vi "Column Headers.vi"(9 "View表":string="[v_runcondition]", 11 "DBLink":string="Driver={ODBC Driver 17 for SQL Server};Server=localhost\\SQLEXPRESS;Database=ZDX201;UID=labview;PWD=Dsa@54137926") -> (1 "資料表欄位名稱":string[](array[string]), 3 "欄位數":i32)   [LabVIEW 2019]
doc: "This VI was put together by AE Steve Karcher with AE Specialist Jonathan Cotton's help."
uses:
  <vilib>/addons/database/Auxilliary.llb/DB Tools Column Info.ctl
  <vilib>/addons/database/Auxilliary.llb/DB Tools DataTypes.ctl
  <vilib>/addons/database/Connection.llb/DB Tools Open Connec (String).vi
  <vilib>/addons/database/Connection.llb/Conn Execute.vi
  <vilib>/addons/database/Recordset.llb/Rec Destroy - Connection.vi
  <vilib>/addons/database/NI_Database_API.lvlib
  <vilib>/addons/database/Recordset.llb/Rec Fetch Recordset Data (R).vi
panel:
  in  "error in (no error)":errorcluster
  out "recordset data":variant[][](array[variant])
  out "error out":errorcluster
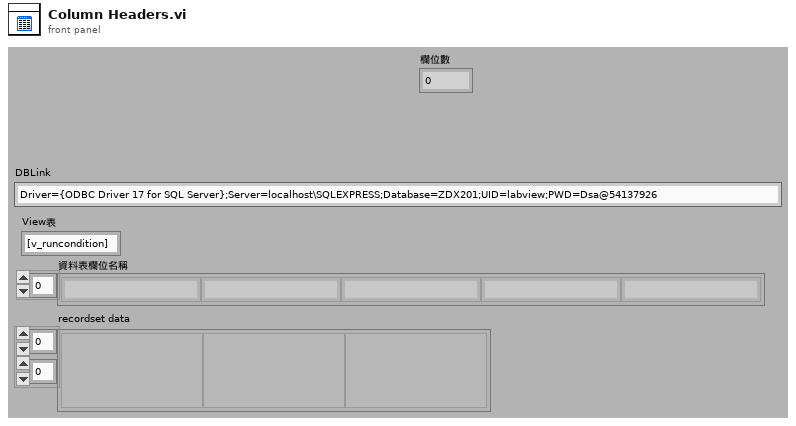
[diagram p1: front panel]
types:
  T1 = cluster{"String":string, "Numeric":i32, "Numeric 2":dbl}
  T2 = typedef "NI_Database_API.lvlib/DB Tools Column Info.ctl" = cluster{"column name":string, "data type":T3, "size":i32, "allow null?":bool}
  T3 = typedef "NI_Database_API.lvlib/DB Tools DataTypes.ctl" = enum16{"String", "Long (I32)", "Single (SGL)", "Double (DBL)", "Date/Time", "Binary"}
  T4 = typedef "NI_Database_API.lvlib/Conn ObjectReference.ctl" = refnum<k1>
  T5 = typedef "NI_Database_API.lvlib/Rec ObjectReference.ctl" = refnum<k1>
  T6 = typedef "NI_Database_API.lvlib/Rec DataMembers.ctl" = cluster{"ADODB._Recordset":refnum<k7>, "Connection":T4}
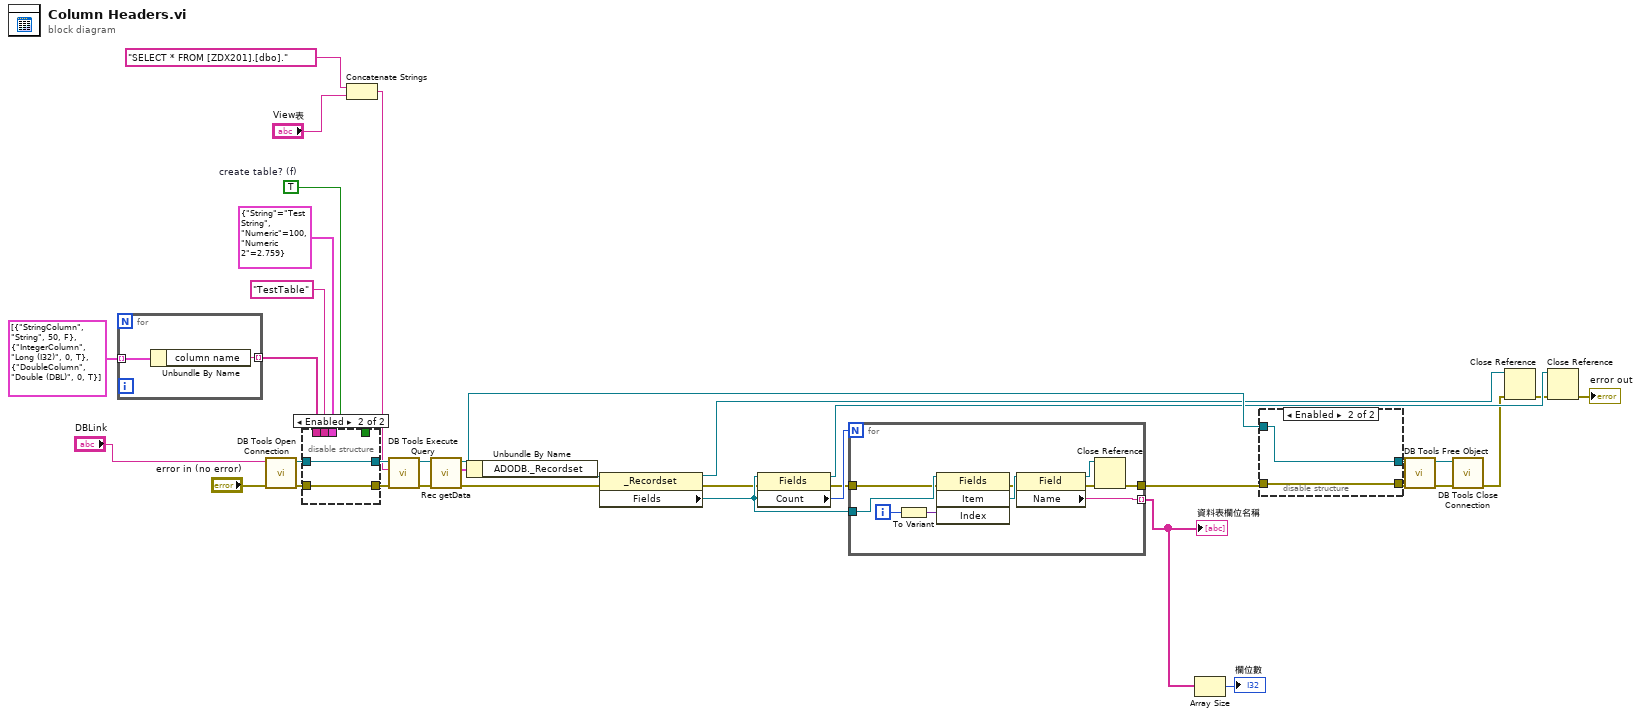
[diagram p0: block diagram]
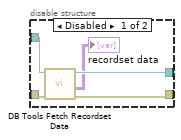
[diagram p2: hidden frame]
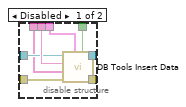
[diagram p3: hidden frame]
diagram:
  w27 = TRUE  # create table? (f)
  n1 = for {
    tunnel: T2[] [{"column name"="StringColumn", "data type"=enum."String", "size"=50, "allow null?"=FALSE}, {"column name"="IntegerColumn", "data type"=enum."Long (I32)", "size"=0, "allow null?"=TRUE}, {"column name"="DoubleColumn", "data type"=enum."Double (DBL)", "size"=0, "allow null?"=TRUE}] ("column information") -> [w38] mode=indexing
    tunnel: [w37] -> w26 mode=indexing
    n2 = Unbundle By Name(w38) -> ("column name"=w37:string)
  }
  n3 = call-poly <vilib>:"DB Tools Open Connection.vi"("error in (no error)"="error in (no error)", "connection information"="DBLink") -> ("error out"=w30:errorcluster, "connection reference"=w31:T4)  [unwired: 6 in]
  n4 = disable-structure shown="Enabled" {
    disable-tunnel: "TestTable" ("Table") -> [w46 _]
    disable-tunnel: w31 -> [w45 w48]
    disable-tunnel: w30 -> [w44 w47]
    disable-tunnel: T1 {"String"="Test String", "Numeric"=100, "Numeric 2"=2.759} ("sample data") -> [w43 _]
    disable-tunnel: w27 -> [w42 _]
    disable-tunnel: w26 -> [w41 _]
    disable-tunnel: [w40 w47] -> w25
    disable-tunnel: [w39 w48] -> w24
    frame Disabled {
      n5 = call <vilib>:"DB Tools Insert Data.vi"("create table? (F)"=w42, "data"=w43, "error in (no error)"=w44, "columns"=w41, "table"=w46, "connection reference"=w45) -> ("error out"=w40:errorcluster, "connection reference out"=w39:T4)  [unwired: 4 in]
    }
    frame Enabled {
    }
  }
  n6 = Concatenate Strings("SELECT * FROM [ZDX201].[dbo]." ("SQL query"), "View表") -> (w3:string)
  n7 = call-poly <vilib>:"DB Tools Execute Query.vi"("error in (no error)"=w25, "SQL query"=w3, "connection reference"=w24) -> ("error out"=w21:errorcluster, "recordset reference"=w22:T5)  [unwired: 5 in]
  n8 = call <vilib>:"Rec getData.vi"("error in (no error)"=w21, "recordset reference"=w22) -> ("error out"=w13:errorcluster, "data"=w19:T6, "recordset reference out"=w20:T5)  [unwired: 2 in, 1 out]
  n9 = Unbundle By Name(w19) -> ("ADODB._Recordset"=w18:refnum<k7>)
  n10 = property class="_Recordset"(reference=w18, error in=w13) -> (reference out=w15:refnum<k7>, error out=w12:errorcluster, "Fields"=w14:refnum<k7>)
  n11 = property class="Fields"(reference=w14, error in=w12) -> (reference out=w16:refnum<k7>, error out=w11:errorcluster, "Count"=w17:i32)
  n12 = for {
    N: w17 -> [_]
    tunnel: w14 -> [w58]
    tunnel: [w54] -> w2 mode=indexing
    tunnel: w11 -> [w51]
    tunnel: [w49] -> w10
    i -> [w57]
    n13 = To Variant(anything=w57) -> (Variant=w56:variant)
    n14 = invoke class="Fields" method="Item"(reference=w58, error in=w51, "Index"=w56) -> (error out=w50:errorcluster, "Item"=w55:refnum<k7>)  [unwired: 1 in, 2 out]
    n15 = property class="Field"(reference=w55, error in=w50) -> (reference out=w52:refnum<k7>, error out=w53:errorcluster, "Name"=w54:string)
    n16 = Close Reference(reference=w52, error in (no error)=w53) -> (error out=w49:errorcluster)
  }
  "資料表欄位名稱" <- w2
  n17 = Array Size(array=w2) -> (size(s)=→"欄位數":i32)
  n18 = disable-structure shown="Enabled" {
    disable-tunnel: [w63 w65] -> w36
    disable-tunnel: [w62 w64] -> w34
    disable-tunnel: w20 -> [w60 w65]
    disable-tunnel: w10 -> [w59 w64]
    frame Disabled {
      n19 = call-poly <vilib>:"DB Tools Fetch Recordset Data.vi"("error in (no error)"=w59, "recordset reference"=w60) -> ("error out"=w62:errorcluster, "recordset data"=→"recordset data":variant[][], "recordset reference out"=w63:T5)  [unwired: 3 in]
    }
    frame Enabled {
    }
  }
  n20 = call-poly <vilib>:"DB Tools Free Object.vi"("error in (no error)"=w34, "recordset reference"=w36) -> ("error out"=w33:errorcluster, "connection reference"=w35:T4)  [unwired: 8 in]
  n21 = call <vilib>:"DB Tools Close Connection.vi"("error in (no error)"=w33, "connection reference"=w35) -> ("error out"=w9:errorcluster)  [unwired: 5 in]
  n22 = Close Reference(reference=w15, error in (no error)=w9) -> (error out=w8:errorcluster)
  n23 = Close Reference(reference=w16, error in (no error)=w8) -> (error out=→"error out":errorcluster)
